vi "例5.13  生成一段随机信号.vi"() -> ()   [LabVIEW 2017]
panel:
  out "波形图":waveform(dbl)(graph)
  out "输出波形":waveform(dbl)
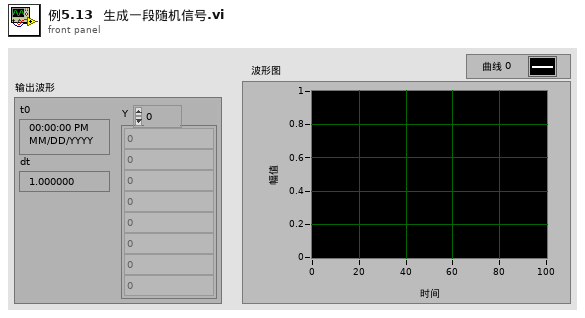
[diagram p1: front panel]
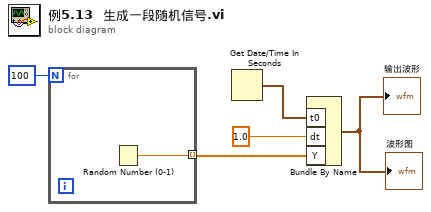
[diagram p0: block diagram]
diagram:
  n1 = for {
    N: 100 -> [_]
    tunnel: [w6] -> w4 mode=indexing
    n2 = Random Number (0-1)() -> (number: 0 to 1=w6:dbl)
  }
  n3 = Get Date/Time In Seconds() -> (seconds since 1Jan1904=w2:timestamp)
  n4 = Bundle By Name("t0"=w2, "dt"=1.0, "Y"=w4) -> (→"输出波形" →"波形图":waveform(dbl))  [unwired: 1 in]
